vi "myFGV.vi"(7 "P/S?":bool, 9 "String 2":string, 10 "Numeric 2":dbl format="%#_13g", 11 "Boolean 2":bool) -> (1 "String":string, 2 "Numeric":dbl, 3 "Boolean":bool)   [LabVIEW 2020]
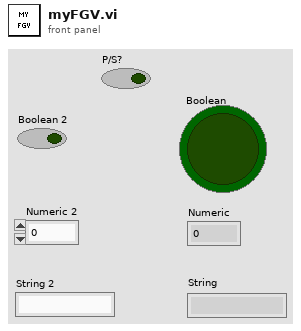
[diagram p1: front panel]
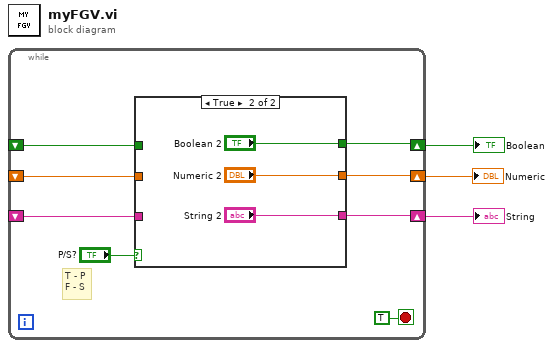
[diagram p0: block diagram]
diagram:
  n1 = while {
    shift-right: [w10] -> w3
    shift-left: _ -> [w6]
    shift-right: [w9] -> w2
    shift-left: _ -> [w5]
    shift-right: [w8] -> w1
    shift-left: _ -> [w4]
    stop <- TRUE stop-if-true
    # "T - P\nF - S"
    n2 = case shown="True" "P/S?" {
      tunnel: [w14 "Boolean 2"] -> w10
      tunnel: [w13 "Numeric 2"] -> w9
      tunnel: [w12 "String 2"] -> w8
      tunnel: w6 -> [w14 _]
      tunnel: w5 -> [w13 _]
      tunnel: w4 -> [w12 _]
      frame False {
      }
      frame True {
      }
    }
  }
  "Boolean" <- w3
  "Numeric" <- w2
  "String" <- w1
